vi "niDTS WLAN DSSS Tx Test Fetch Results.vi"(0 "Dummy Test Handle in":T16, 11 "error in (no error)":errorcluster) -> (4 "Dummy Test Handle out":T16, 8 "Results":T1 {"OBW"."Stop Frequency (Hz)" format="%#_4p"; "OBW"."Start Frequency (Hz)" format="%#_4p"; "OBW"."OBW (Hz)" format="%#_4p"}, 15 "error out":errorcluster)   [LabVIEW 2014, in "niDTS WLAN.lvlib"]
uses:
  niDTS WLAN.lvlib
  Tx Test/Includes/niDTS WLAN Tx Test INC Handle.ctl
  Tx Test/Objects/BASE_class/niDTS WLAN Tx Test.lvclass
  Tx Test/Includes/niDTS WLAN Tx Test INC DSSS Results.ctl
  Tx Test/Includes/niDTS WLAN Tx Test INC DSSS MOD EVM Results.ctl
  Includes/Results/niDTS WLAN DSSS Tx RES EVM ALL.ctl
  Includes/Results/niDTS WLAN DSSS Tx RES EVM RMS.ctl
  Tx Test/Includes/niDTS WLAN Tx Test INC TXP Results.ctl
  Tx Test/Includes/niDTS WLAN Tx Test INC TXP Result SINGLE.ctl
  Tx Test/Includes/niDTS WLAN Tx Test INC OBW Results.ctl
  Instrument/INSTR TX/Results/niDTS WLAN INSTR TX INC SEM Results.ctl
  Instrument/INSTR TX/Results/niDTS WLAN INSTR TX INC SEM FSEGemts Results.ctl
  Tx Test/Includes/Results/niDTS Tx RES INC SEM FSEGemts.ctl
  Instrument/INSTR TX/Results/niDTS WLAN INSTR TX INC SEM MARGin Results.ctl
  Tx Test/Includes/Results/niDTS Tx RES INC SEM Margin.ctl
  Tx Test/Includes/niDTS WLAN Tx Test INC DSSS MOD Impairments Results.ctl
  Includes/Results/niDTS WLAN DSSS Tx Impairmentsctl.ctl
  Includes/Results/niDTS WLAN DSSS Tx PowerRamp.ctl
  Instrument/INSTR TX/niDTS WLAN INSTR TX.lvclass
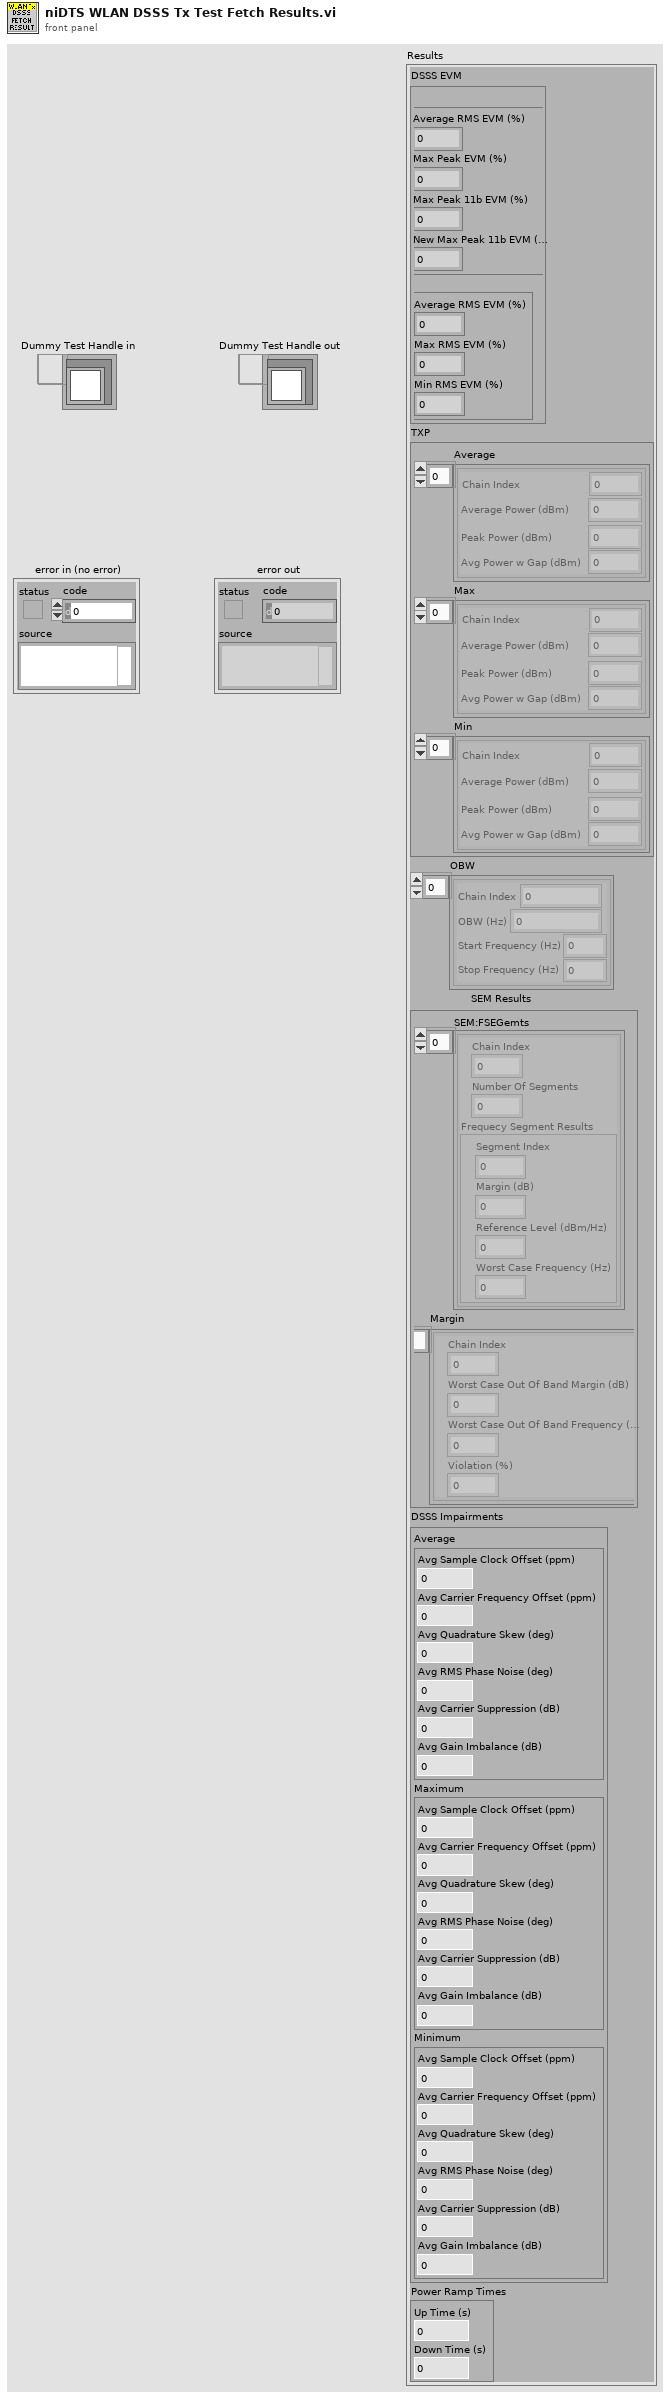
[diagram p1: front panel]
types:
  T1 = typedef "niDTS WLAN.lvlib/niDTS WLAN Tx Test INC DSSS Results.ctl" = cluster{"DSSS EVM":T2, "TXP":T5, "OBW":T7[], "SEM Results":T8, "DSSS Impairments":T13, "Power Ramp Times":T15}
  T2 = typedef "niDTS WLAN.lvlib/niDTS WLAN Tx Test INC DSSS MOD EVM Results.ctl" = cluster{"All":T3, "RMS":T4}
  T3 = typedef "niDTS WLAN.lvlib/niDTS WLAN DSSS Tx RES EVM ALL.ctl" = cluster{"Average RMS EVM (%)":dbl, "Max Peak EVM (%)":dbl, "Max Peak 11b EVM (%)":dbl, "New Max Peak 11b EVM (%)":dbl}
  T4 = typedef "niDTS WLAN.lvlib/niDTS WLAN DSSS Tx RES EVM RMS.ctl" = cluster{"Average RMS EVM (%)":dbl, "Max RMS EVM (%)":dbl, "Min RMS EVM (%)":dbl}
  T5 = typedef "niDTS WLAN.lvlib/niDTS WLAN Tx Test INC TXP Results.ctl" = cluster{"Average":T6[], "Max":T6[], "Min":T6[]}
  T6 = typedef "niDTS WLAN.lvlib/niDTS WLAN Tx Test INC TXP Result SINGLE.ctl" = cluster{"Chain Index":dbl, "Average Power (dBm)":dbl, "Peak Power (dBm)":dbl, "Avg Power w Gap (dBm)":dbl}
  T7 = typedef "niDTS WLAN.lvlib/niDTS WLAN Tx Test INC OBW Results.ctl" = cluster{"Chain Index":dbl, "OBW (Hz)":dbl, "Start Frequency (Hz)":dbl, "Stop Frequency (Hz)":dbl}
  T8 = typedef "niDTS WLAN.lvlib/niDTS WLAN INSTR TX.lvclass/niDTS WLAN INSTR TX INC SEM Results.ctl" = cluster{"SEM:FSEGemts":T9, "Margin":T11}
  T9 = typedef "niDTS WLAN.lvlib/niDTS WLAN INSTR TX.lvclass/niDTS WLAN INSTR TX INC SEM FSEGemts Results.ctl" = T10[]
  T10 = typedef "niDTS WLAN.lvlib/niDTS Tx RES INC SEM FSEGemts.ctl" = cluster{"Chain Index":i32, "Number Of Segments":i32, "Frequecy Segment Results":cluster{"Segment Index":i32, "Margin (dB)":dbl, "Reference Level (dBm/Hz)":dbl, "Worst Case Frequency (Hz)":dbl}}
  T11 = typedef "niDTS WLAN.lvlib/niDTS WLAN INSTR TX.lvclass/niDTS WLAN INSTR TX INC SEM MARGin Results.ctl" = T12[]
  T12 = typedef "niDTS WLAN.lvlib/niDTS Tx RES INC SEM Margin.ctl" = cluster{"Chain Index":i32, "Worst Case Out Of Band Margin (dB)":dbl, "Worst Case Out Of Band Frequency (Hz)":dbl, "Violation (%)":dbl}
  T13 = typedef "niDTS WLAN.lvlib/niDTS WLAN Tx Test INC DSSS MOD Impairments Results.ctl" = cluster{"Average":T14, "Maximum":T14, "Minimum":T14}
  T14 = typedef "niDTS WLAN.lvlib/niDTS WLAN DSSS Tx Impairmentsctl.ctl" = cluster{"Avg Sample Clock Offset (ppm)":dbl, "Avg Carrier Frequency Offset (ppm)":dbl, "Avg Quadrature Skew (deg)":dbl, "Avg RMS Phase Noise (deg)":dbl, "Avg Carrier Suppression (dB)":dbl, "Avg Gain Imbalance (dB)":dbl}
  T15 = typedef "niDTS WLAN.lvlib/niDTS WLAN DSSS Tx PowerRamp.ctl" = cluster{"Up Time (s)":dbl, "Down Time (s)":dbl}
  T16 = typedef "niDTS WLAN.lvlib/niDTS WLAN Tx Test INC Handle.ctl" = refnum<data-value>
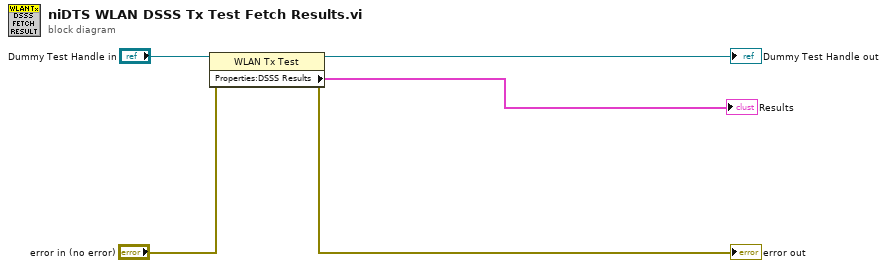
[diagram p0: block diagram]
diagram:
  n1 = property class="WLAN Tx Test"(reference="Dummy Test Handle in", error in="error in (no error)") -> (reference out=→"Dummy Test Handle out":T16, error out=→"error out":errorcluster, "Properties:DSSS Results"=→"Results":T1)
